vi "Add (SubVI).vi"(11 "Input Add":i32[](array[numeric])=[2, 2, 4, 4]) -> (1 "Score 2":i32, 2 "Output Add 2":i32[](array[numeric])=[0, 3, 2, 1], 3 "Add changed?":bool)   [LabVIEW 2020]
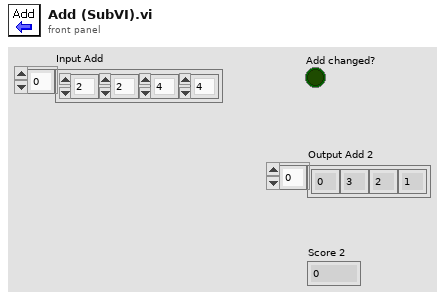
[diagram p1: front panel]
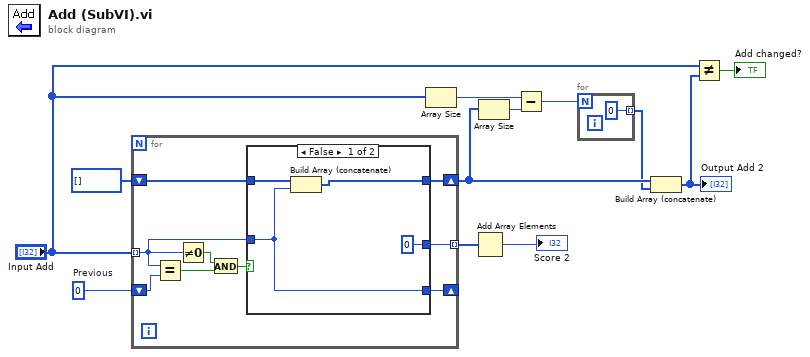
[diagram p0: block diagram]
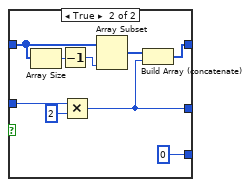
[diagram p2: hidden frame]
diagram:
  w3 = 0  # Previous
  n1 = for {
    shift-right: [w19] -> w7
    shift-left: i32[] [] ("Array") -> [w20]
    tunnel: "Input Add" -> [w14] mode=indexing
    shift-right: [w18] -> _
    shift-left: w3 -> [w21]
    tunnel: [w13] -> w8 mode=indexing
    n2 = Equal?(x=w14, y=w21) -> (x = y?=w17:bool)
    n3 = Not Equal To 0?(x=w14) -> (x != 0?=w15:bool)
    n4 = And(x=w15, y=w17) -> (x .and. y?=w16:bool)
    n5 = case shown="False" w16 {
      tunnel: w20 -> [w25 w28]
      tunnel: w14 -> [w23 w34]
      tunnel: [w24 w32] -> w19
      tunnel: [w23 0 ("Previous")] -> w18
      tunnel: [0 w26] -> w13
      frame False {
        n6 = Build Array (concatenate)(w25, w23) -> (w24:i32[])
      }
      frame True {
        n7 = Array Size(array=w28) -> (size(s)=w29:i32)
        n8 = Decrement(x=w29) -> (x-1=w27:i32)
        n9 = Multiply(x=w34, y=2) -> (x*y=w26:i32)
        n10 = Array Subset(array=w28, length=w27) -> (w30:i32[])  [unwired: 1 in]
        n11 = Build Array (concatenate)(w30, w26) -> (w32:i32[])
      }
    }
  }
  n12 = Array Size(array="Input Add") -> (size(s)=w6:i32)
  n13 = Add Array Elements(numeric array=w8) -> (sum=→"Score 2":i32)
  n14 = Array Size(array=w7) -> (size(s)=w4:i32)
  n15 = Subtract(x=w6, y=w4) -> (x-y=w9:i32)
  n16 = for {
    N: w9 -> [_]
    tunnel: [0 ("Numeric")] -> w5 mode=indexing
  }
  n17 = Build Array (concatenate)(w7, w5) -> (w11:i32[])
  "Output Add 2" <- w11
  n18 = Not Equal?(x="Input Add", y=w11) -> (x != y?=→"Add changed?":bool)
